vi "Calibration Parameters.vi"(6 "Standard Calibration (F:Off)":bool, 8 "error in (no error)":errorcluster, 9 "Short Calibration (F:Off)":bool, 10 "Open Calibration (F:Off)":bool, 11 "VISA resource name":refnum<visa-resource-name>) -> (0 "error out":errorcluster, 3 "VISA resource name out":refnum<visa-resource-name>)   [LabVIEW 2010, in "Agilent 4194.lvlib"]
doc: "This function sets the basic calibration parameters or activates normalization."
uses:
  <instrlib>/Agilent 4194/Agilent 4194.lvlib
panel:
  # "On\nOff"
  # "On\nOff"
  # "On\nOff"
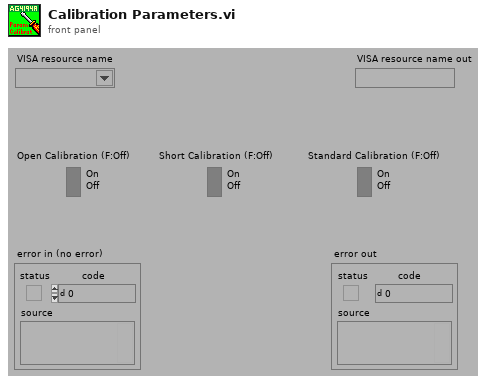
[diagram p1: front panel]
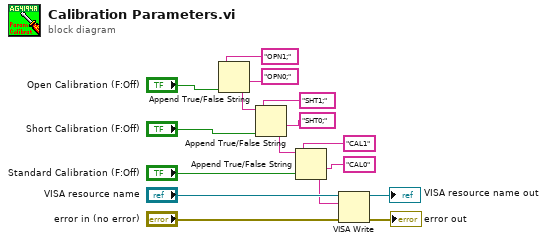
[diagram p0: block diagram]
diagram:
  n1 = Append True/False String(1:"Open Calibration (F:Off)", 2:"OPN0;" ("true string"), 3:"OPN1;" ("true string")) -> (0:w3:string)  [unwired: 1 in]
  n2 = Append True/False String(1:"Short Calibration (F:Off)", 2:"SHT0;" ("true string"), 3:"SHT1;" ("true string"), 4:w3) -> (0:w2:string)
  n3 = Append True/False String(1:"Standard Calibration (F:Off)", 2:"CAL0" ("true string"), 3:"CAL1" ("true string"), 4:w2) -> (0:w1:string)
  n4 = VISA Write(VISA resource name="VISA resource name", write buffer=w1, error in (no error)="error in (no error)") -> (VISA resource name out=→"VISA resource name out":refnum<visa-resource-name>, error out=→"error out":errorcluster)  [unwired: 1 out]
